vi "Get Paths.vi"(8 "error in (no error)":errorcluster) -> (0 "error out":errorcluster, 2 "actual path":path, 3 "approved path":path)   [LabVIEW 2020]
doc: "Generates 2 absolute paths based on the name of the calling unit test.\n\nname_of_unit_test.approved\nname_of_unit_test.actual"
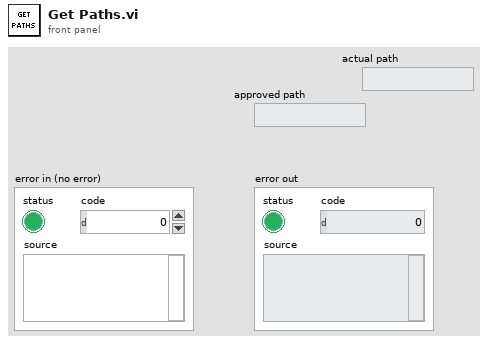
[diagram p1: front panel]
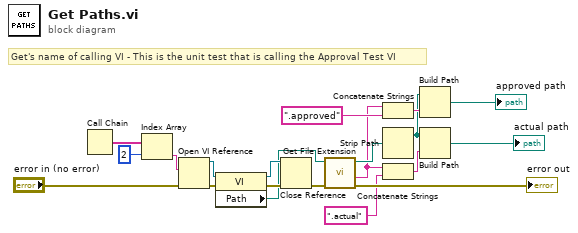
[diagram p0: block diagram]
diagram:
  # "Get's name of calling VI - This is the unit test that is calling the Approval Test VI"
  n1 = Call Chain() -> (call chain=w9:string[])
  n2 = Index Array(array=w9, index=2) -> (element=w11:string)
  n3 = Open VI Reference(vi path=w11, error in (no error)="error in (no error)") -> (vi reference=w12:refnum<vi>, error out=w13:errorcluster)  [unwired: 4 in]
  n4 = property on="Property Node" class="VI"(reference=w12, error in=w13) -> (reference out=w16:refnum<vi>, error out=w15:errorcluster, "Path"=w14:path)
  n5 = Close Reference(reference=w16, error in (no error)=w15) -> (error out=w17:errorcluster)
  n6 = call <vilib>:"Get File Extension.vi"("error in (no error)"=w17, "file"=w14) -> ("error out"=→"error out":errorcluster, "filename without extension"=w1:string, "dup file"=w6:path)  [unwired: 5 in, 2 out]
  n7 = Concatenate Strings(w1, ".approved" ("string")) -> (w8:string)
  n8 = Strip Path(path=w6) -> (stripped path=w3:path)  [unwired: 1 out]
  n9 = Concatenate Strings(w1, ".actual" ("string")) -> (w4:string)
  n10 = Build Path(base path=w3, name or relative path=w8) -> (appended path=→"approved path":path)
  n11 = Build Path(base path=w3, name or relative path=w4) -> (appended path=→"actual path":path)
